vi "Example.vi"() -> ()   [LabVIEW 2013, in "TektronixDPO_PhysicalDevice.lvclass"]
uses:
  TektronixDPO_PhysicalDevice.lvclass
  shared/Typdefs/Choice80.ctl
  shared/Typdefs/Choice78.ctl
  shared/Typdefs/Choice11.ctl
  shared/Typdefs/Choice79.ctl
  TektronixDPO_PhysicalDevice.lvclass/TektronixDPO_PhysicalDevice.ctl
panel:
  out "ActiveChannel":T5 {"Channel" items=["Channel 1", "Channel 2", "Channel 3", "Channel 4", "Math", "Reference 1", "Reference 2", "Reference 3", "Reference 4", "Bus 1", "Bus 2"]}
  out "error out":errorcluster
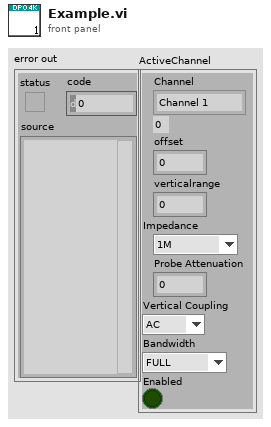
[diagram p1: front panel]
types:
  T1 = typedef "Choice80.ctl" = u16
  T2 = typedef "Choice78.ctl" = enum16{"1M", "75", "50"}
  T3 = typedef "Choice11.ctl" = enum16{"AC", "DC", "Ground"}
  T4 = typedef "Choice79.ctl" = enum16{"FULL", "250 MHz", "150 MHz", "20 MHz"}
  T5 = cluster{"Channel":T1, "offset":dbl, "verticalrange":dbl, "Impedance":T2, "Probe Attenuation":dbl, "Vertical Coupling":T3, "Bandwidth":T4, "Enabled":bool}
  T6 = cluster{"Channel":T1, "offset":dbl, "verticalrange":dbl, "Impedance":T2, "probeattenuation":dbl, "coupling":T3, "bandwidth":T4, "channelenabled":bool}
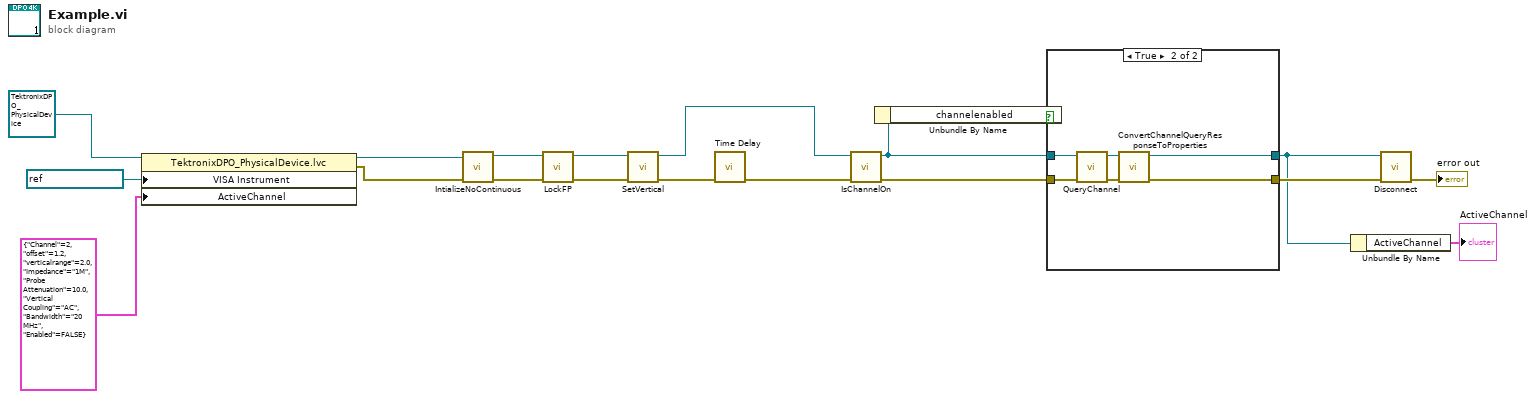
[diagram p0: block diagram]
diagram:
  n1 = property class="TektronixDPO_PhysicalDevice.lvc"(reference=refnum<class "TektronixDPO_PhysicalDevice.lvclass"> refnum ("TektronixDPO_PhysicalDevice.lvclass"), "VISA Instrument"=refnum<visa-resource-name> "P2_TekScope", "ActiveChannel"=T5 {"Channel"=2, "offset"=1.2, "verticalrange"=2.0, "Impedance"=enum."1M", "Probe Attenuation"=10.0, "Vertical Coupling"=enum."AC", "Bandwidth"=enum."20 MHz", "Enabled"=FALSE}) -> (reference out=w17:refnum<class "TektronixDPO_PhysicalDevice.lvclass">, error out=w15:errorcluster)  [unwired: 1 in]
  n2 = call "IntializeNoContinuous.vi"("error in (no error)"=w15, "TektronixDPO_PhysicalDevice in"=w17) -> ("error out"=w11:errorcluster, "TektronixDPO_PhysicalDevice out"=w10:refnum<class "TektronixDPO_PhysicalDevice.lvclass">)  [unwired: 8 in]
  n3 = call "LockFP.vi"("error in (no error)"=w11, "TektronixDPO_PhysicalDevice in"=w10) -> ("error out"=w9:errorcluster, "TektronixDPO_PhysicalDevice out"=w8:refnum<class "TektronixDPO_PhysicalDevice.lvclass">)  [unwired: 8 in]
  n4 = call "SetVertical.vi"("error in (no error)"=w9, "TektronixDPO in"=w8) -> ("error out"=w13:errorcluster, "TektronixDPO_PhysicalDevice.lvclass"=w6:refnum<class "TektronixDPO_PhysicalDevice.lvclass">)  [unwired: 8 in]
  n5 = call "Time Delay"("error in (no error)"=w13) -> ("error out"=w7:errorcluster)  [unwired: 10 in]
  n6 = call "IsChannelOn.vi"("error in (no error)"=w7, "TektronixDPO_PhysicalDevice in"=w6) -> ("error out"=w4:errorcluster, "TektronixDPO_PhysicalDevice out"=w3:refnum<class "TektronixDPO_PhysicalDevice.lvclass">)  [unwired: 8 in]
  n7 = Unbundle By Name(w3) -> ("channelenabled"=w5:bool)
  n8 = case shown="True" w5 {
    tunnel: [w21 w27] -> w2
    tunnel: [w20 w26] -> w14
    tunnel: w4 -> [w20 w24]
    tunnel: w3 -> [w21 w23]
    frame False {
    }
    frame True {
      n9 = call "QueryChannel.vi"("error in (no error)"=w24, "TektronixDPO_PhysicalDevice in"=w23) -> ("error out"=w25:errorcluster, "TektronixDPO_PhysicalDevice out"=w22:refnum<class "TektronixDPO_PhysicalDevice.lvclass">)  [unwired: 8 in]
      n10 = call-dynamic "ConvertChannelQueryResponseToProperties.vi"("error in (no error)"=w25, "TektronixDPO_PhysicalDevice.lvclass"=w22) -> ("error out"=w26:errorcluster, "TektronixDPO_PhysicalDevice.lvclassOut"=w27:refnum<class "TektronixDPO_PhysicalDevice.lvclass">)  [unwired: 8 in]
    }
  }
  n11 = Unbundle By Name(w2) -> ("ActiveChannel"=→"ActiveChannel":T6)
  n12 = call "Disconnect.vi"("error in (no error)"=w14, "TektronixDPO_PhysicalDevice in"=w2) -> ("error out"=→"error out":errorcluster)  [unwired: 9 in]
